vi "readPath.vi"(8 "error in (no error)":errorcluster, 10 "file (use dialog)":path, 11 "regular expression":string) -> (0 "error out":errorcluster, 2 "path":path, 3 "file or folder exists?":bool)   [LabVIEW 2020]
panel:
  out "valInt":i32
  out "vlafSGL":dbl
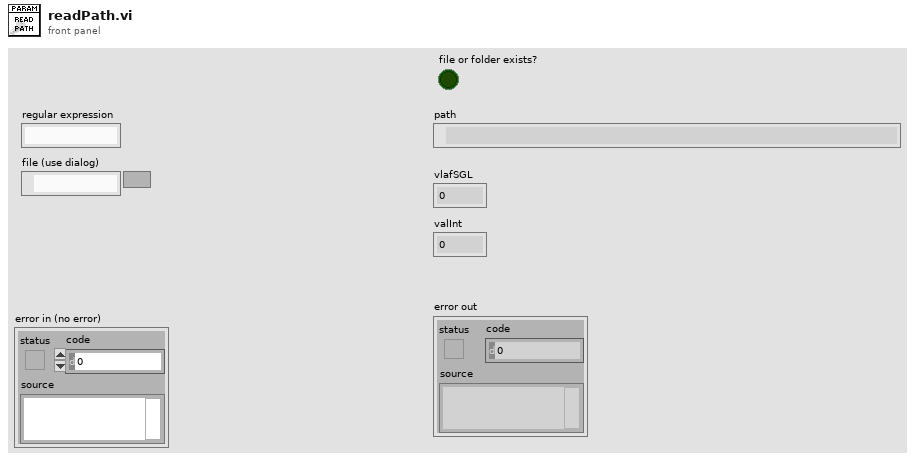
[diagram p1: front panel]
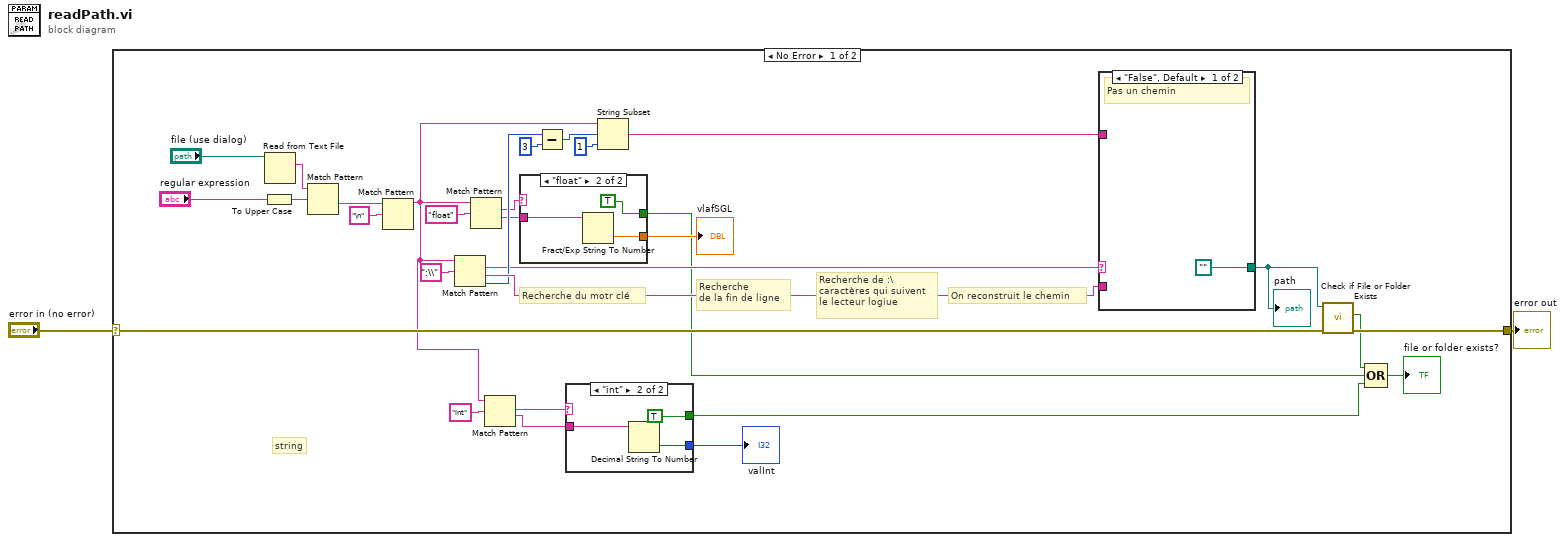
[diagram p0: block diagram]
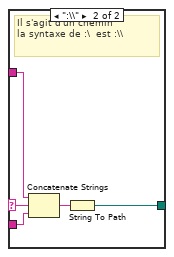
[diagram p4: hidden frame]
diagram:
  n1 = case shown="No Error" "error in (no error)" {
    selector: "error in (no error)" -> [w19 w45]
    tunnel: [w20 w45] -> w2
    frame No Error {
      # "string"
      # "On reconstruit le chemin"
      # "Recherche de :\\\ncaractères qui suivent \nle lecteur logiue"
      # "Recherche \nde la fin de ligne"
      # "Recherche du motr clé"
      n2 = To Upper Case(1:"regular expression") -> (0:w22:string)
      n3 = Read from Text File(file (use dialog)="file (use dialog)") -> (text=w31:string)  [unwired: 3 in, 3 out]
      n4 = Match Pattern(string=w31, regular expression=w22) -> (after substring=w29:string)  [unwired: 1 in, 3 out]
      n5 = Match Pattern(string=w29, regular expression="\n") -> (before substring=w10:string)  [unwired: 1 in, 3 out]
      n6 = Match Pattern(string=w10, regular expression=":\\") -> (match substring=w16:string, after substring=w26:string, offset past match=w25:i32)  [unwired: 1 in, 1 out]
      n7 = Match Pattern(string=w10, regular expression="float") -> (match substring=w13:string, after substring=w14:string)  [unwired: 1 in, 2 out]
      n8 = Match Pattern(string=w10, regular expression="int") -> (match substring=w8:string, after substring=w7:string)  [unwired: 1 in, 2 out]
      n9 = case shown="\"float\"" w13 {
        tunnel: w14 -> [_ w38]
        tunnel: [_ w37] -> w12
        tunnel: [_ TRUE ("file or folder exists?")] -> w3
        frame "False", Default {
        }
        frame "float" {
          n10 = Fract/Exp String To Number(string=w38) -> (number=w37:dbl)  [unwired: 3 in, 1 out]
        }
      }
      "vlafSGL" <- w12
      n11 = Subtract(x=w25, y=3) -> (x-y=w18:i32)
      n12 = case shown="\"int\"" w8 {
        tunnel: w7 -> [_ w35]
        tunnel: [_ w34] -> w9
        tunnel: [_ TRUE ("file or folder exists?")] -> w5
        frame "False", Default {
        }
        frame "int" {
          n13 = Decimal String To Number(string=w35) -> (number=w34:i32)  [unwired: 2 in, 1 out]
        }
      }
      "valInt" <- w9
      n14 = String Subset(string=w10, offset (0)=w18, length (rest)=1 ("length (rest)")) -> (substring=w23:string)
      n15 = case shown="\"False\", Default" w16 {
        selector: w16 -> [_ w40]
        tunnel: w26 -> [_ w44]
        tunnel: w23 -> [_ w43]
        tunnel: [path "" w41] -> w21
        frame "False", Default {
          # "Pas un chemin"
        }
        frame ":\\" {
          # "Il s'agit d'un chemin \nla syntaxe de :\\  est :\\\\"
          n16 = Concatenate Strings(w43, w40, w44) -> (w42:string)
          n17 = String To Path(string=w42) -> (path=w41:path)
        }
      }
      "path" <- w21
      n18 = call <vilib>:"Check if File or Folder Exists.vi"("error in (no error)"=w19, "path"=w21) -> ("error out"=w20:errorcluster, "file or folder exists?"=w4:bool)  [unwired: 7 in, 1 out]
      n19 = Compound Arithmetic op=OR(w4, w3, w5) -> (→"file or folder exists?":bool)
    }
    frame Error {
    }
  }
  "error out" <- w2
